vi "Draw整体图.vi"() -> ()   [LabVIEW 2014]
panel:
  in  "Gimp":bool
  in  "Fill":bool
  in  "Edit":bool
  in  "Draw":bool
  in  "Cw":bool
  in  "Contour":bool
  in  "Colors":bool
  in  "Colorize":bool
  in  "Choose":bool
  in  "Ccw":bool
  in  "Blend":bool
  in  "Rotate":bool
  in  "Pencil":bool
  in  "Pen":bool
  in  "Paint":bool
  in  "Modeler":bool
  in  "Measure":bool
  in  "Line":bool
  in  "Graphics":bool
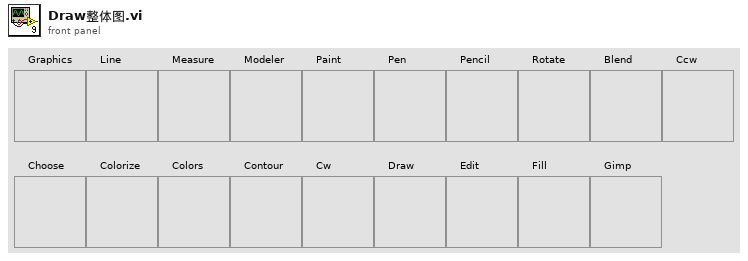
[diagram p1: front panel]
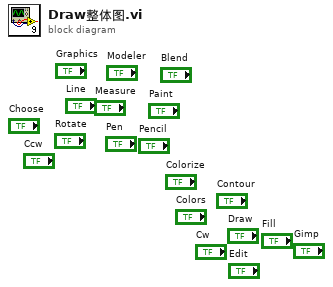
[diagram p0: block diagram]
diagram:
